vi "Get Error Description.vi"(8 "error in":errorcluster, 11 "error code":i32) -> (0 "error out":errorcluster, 3 "error description":string)   [LabVIEW 2020, in "AIM ARINC 429 Hardware API.lvlib"]
uses:
  AIM ARINC 429 Hardware API.lvlib
  <instrlib>/_AIM 429/AIM429LV.lvlib
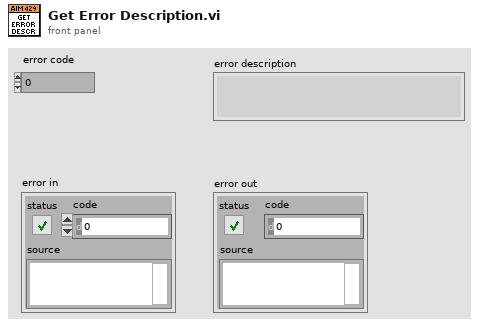
[diagram p1: front panel]
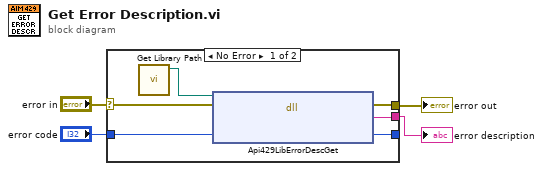
[diagram p0: block diagram]
diagram:
  n1 = case shown="No Error" "error in" {
    selector: "error in" -> [w10 _]
    tunnel: "error code" -> [w9 _]
    tunnel: [w8 _] -> w2
    tunnel: [w7 _] -> _
    tunnel: [w6 _] -> w1
    frame No Error {
      n2 = call <instrlib>:"Get Library Path.vi"() -> ("GlobalDLLPath"=w5:path)  [unwired: 11 in]
      n3 = dll-call lib="api_civ.9.dll" fn="Api429LibErrorDescGet" ("Ai429.dll:Api429CmdTxMajFrameInstCvi")(path in=w5, error in=w10, "ul_ErrorCode"=w9) -> (error out=w6:errorcluster, "name"=w8:string, "ul_ErrorCode"=w7:i32)  [unwired: 1 in, 1 out]
    }
    frame Error {
    }
  }
  "error description" <- w2
  "error out" <- w1
